vi "Register gRPC Methods and Messages.vi"(8 "error in (no error)":errorcluster, 10 "gRPC ID in":T1, 11 "MeasurementServiceV2 in":refnum<class "MeasurementServiceV2.lvclass">) -> (0 "error out":errorcluster, 2 "gRPC ID out":T1, 3 "MeasurementServiceV2 out":refnum<class "MeasurementServiceV2.lvclass">)   [LabVIEW 2020, in "MeasurementLink Measurement Server.lvlib" / "MeasurementServiceV2.lvclass"]
uses:
  MeasurementServiceV2.lvclass
  <vilib>/gRPC/LabVIEW gRPC Library/Shared/grpcId.ctl
  MeasurementServiceV2.lvclass/MeasurementServiceV2.ctl
  MeasurementLink Measurement Service Base V2/RPC Service/MeasurementService/MeasurementServiceBaseV2.lvclass
  MeasurementLink Measurement Service Base V2/MeasurementLink Measurement Service Base V2.lvlib
  <vilib>/gRPC/LabVIEW gRPC Library/grpc-lvsupport-release.lvlib
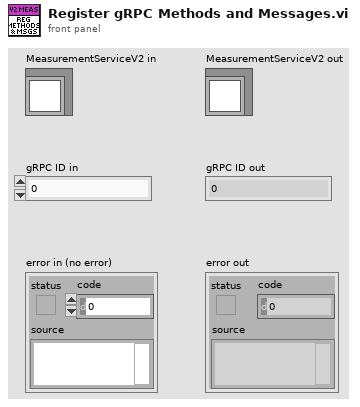
[diagram p1: front panel]
types:
  T1 = typedef "grpc-lvsupport-release.lvlib/grpcId.ctl" = u64
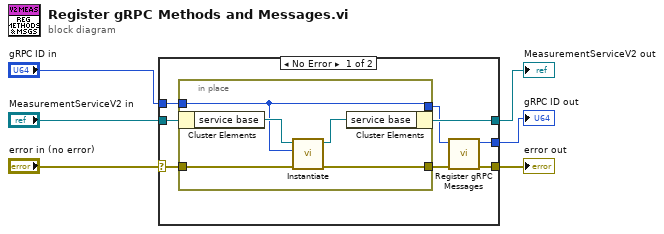
[diagram p0: block diagram]
diagram:
  n1 = case shown="No Error" "error in (no error)" {
    selector: "error in (no error)" -> [w9 w22]
    tunnel: [w13 w22] -> w5
    tunnel: [w10 w21] -> w3
    tunnel: "MeasurementServiceV2 in" -> [w11 w21]
    tunnel: "gRPC ID in" -> [w8 w20]
    tunnel: [w14 w20] -> w1
    frame No Error {
      n2 = in-place {
        in-place-border: [w17] -> w12
        in-place-border: w9 -> [w16]
        in-place-border: w8 -> [w15]
        in-place-border: [w15] -> w7
        n3 = in-place-cluster #1(w11) -> ("service base"=w19:refnum<class "MeasurementServiceBaseV2.lvclass">)
        n4 = call-dynamic "Instantiate.vi"("error in"=w16, "gRPCid"=w15, "iService"=w19) -> ("error out"=w17:errorcluster, "iService"=w18:refnum<class "MeasurementServiceBaseV2.lvclass">)  [unwired: 7 in]
        n5 = in-place-cluster #1("service base"=w18) -> (w10:refnum<class "MeasurementServiceV2.lvclass">)
      }
      n6 = call "Register gRPC Messages.vi"("error in (no error)"=w12, "gRPC ID"=w7) -> ("error out"=w13:errorcluster, "gRPC ID Out"=w14:T1)  [unwired: 8 in]
    }
    frame Error {
    }
  }
  "error out" <- w5
  "MeasurementServiceV2 out" <- w3
  "gRPC ID out" <- w1
